vi "Tosca-Init AI Processing.vi"(0 "Queue data":T2) -> (4 "state":T1)   [LabVIEW 2020]
uses:
  Typedefs/Tosca-AI Control Queue Data.ctl
  Typedefs/Tosca-AI.ctl
  Typedefs/Tosca-AI Plot State.ctl
  epl-vi-lib/Connection VIs/Type Defs/CM-IO Type.ctl
  Sub VIs/Tosca-Globals.vi
  epl-vi-lib/Utility VIs/Array Manipulation VIs/Sort and Index (string).vi
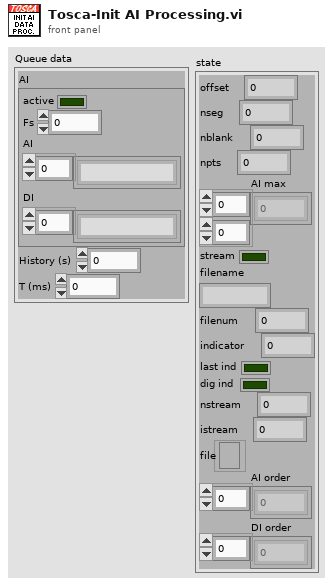
[diagram p1: front panel]
types:
  T1 = typedef "Tosca-AI Plot State.ctl" = cluster{"offset":i32, "nseg":i32, "nblank":i32, "npts":i32, "AI max":dbl[][], "stream":bool, "filename":string, "filenum":i32, "indicator":i32, "last ind":bool, "dig ind":bool, "nstream":i32, "istream":i32, "file":refnum<file>, "AI order":i32[], "DI order":i32[]}
  T2 = typedef "Tosca-AI Control Queue Data.ctl" = cluster{"AI":T3, "History (s)":dbl, "T (ms)":dbl}
  T3 = typedef "Tosca-AI.ctl" = cluster{"active":bool, "Fs":dbl, "AI":string[], "DI":string[]}
  T4 = typedef "CM-IO Type.ctl" = enum16{"Analog Outputs", "Analog Inputs", "Digital Outputs", "Digital Inputs"}
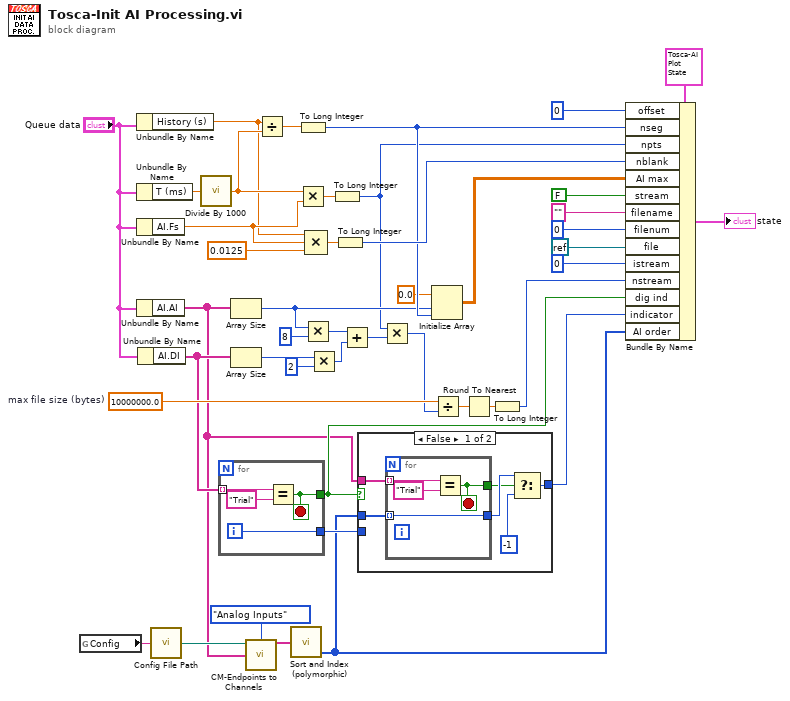
[diagram p0: block diagram]
diagram:
  w15 = 10000000.0  # max file size (bytes)
  n1 = global read "Tosca-Globals.vi" "Config"() -> (w1:string)
  n2 = Unbundle By Name("Queue data") -> ("History (s)"=w31:dbl)
  n3 = Unbundle By Name("Queue data") -> ("T (ms)"=w30:dbl)
  n4 = Unbundle By Name("Queue data") -> ("AI.Fs"=w39:dbl)
  n5 = Unbundle By Name("Queue data") -> ("AI.AI"=w3:string[])
  n6 = Unbundle By Name("Queue data") -> ("AI.DI"=w10:string[])
  n7 = call "Config File Path.vi"("AppName"=w1) -> ("Default config file name"=w6:path)
  n8 = call "Divide By 1000.vi"("X"=w30) -> ("X/1000"=w35:dbl)
  n9 = for {
    tunnel: w10 -> [w48] mode=indexing
    tunnel: [w46] -> w9
    tunnel: [w45] -> w7
    i -> [w46]
    stop <- w45 stop-if-true
    n10 = Equal?(x=w48, y="Trial") -> (x = y?=w45:bool)
  }
  n11 = Array Size(array=w3) -> (size(s)=w23:i32)
  n12 = Array Size(array=w10) -> (size(s)=w21:i32)
  n13 = call "CM-Endpoints to Channels.vi"("Path"=w6, "IO Type"=CM-IO_Type."Analog Inputs", "Requested Endpoints"=w3) -> ("IO Channels"=w4:string[])  [unwired: 11 in, 1 out]
  n14 = Divide(x=w31, y=w35) -> (x/y=w44:dbl)
  n15 = call-poly "Sort and Index (polymorphic).vi"("X"=w4) -> ("Index"=w2:i32[])  [unwired: 3 in, 1 out]
  n16 = To Long Integer(number=w44) -> (32bit integer=w34:i32)
  n17 = Multiply(x=w35, y=w39) -> (x*y=w41:dbl)
  n18 = Multiply(x=w23, y=8) -> (x*y=w19:i32)
  n19 = Compound Arithmetic op=MULTIPLY(w31, w39, 0.0125 ("y")) -> (w40:dbl)
  n20 = Multiply(x=w21, y=2) -> (x*y=w18:i32)
  n21 = To Long Integer(number=w41) -> (32bit integer=w16:i32)
  n22 = To Long Integer(number=w40) -> (32bit integer=w37:i32)
  n23 = Add(x=w19, y=w18) -> (x+y=w17:i32)
  n24 = case shown="False" w7 {
    tunnel: w9 -> [_ w59]
    tunnel: w3 -> [w54 _]
    tunnel: [w53 w59] -> w8
    tunnel: w2 -> [w49 _]
    frame False {
      n25 = for {
        tunnel: w54 -> [w58] mode=indexing
        tunnel: [w55] -> w52
        tunnel: [w56] -> w50
        tunnel: w49 -> [w55] mode=indexing
        stop <- w56 stop-if-true
        n26 = Equal?(x=w58, y="Trial") -> (x = y?=w56:bool)
      }
      n27 = Select(t=w52, s=w50, f=-1) -> (s? t:f=w53:i32)
    }
    frame True {
    }
  }
  n28 = Multiply(x=w16, y=w17) -> (x*y=w14:i32)
  n29 = Initialize Array(0.0 ("element"), w23, w34) -> (w32:dbl[][])
  n30 = Divide(x=w15, y=w14) -> (x/y=w13:dbl)
  n31 = Round To Nearest(number=w13) -> (nearest integer value=w12:dbl)
  n32 = To Long Integer(number=w12) -> (32bit integer=w11:i32)
  n33 = Bundle By Name(cluster=T1 {"offset"=0, "nseg"=0, "nblank"=0, "npts"=0, "AI max"=[], "stream"=FALSE, "filename"="", "filenum"=0, "indicator"=0, "last ind"=FALSE, "dig ind"=FALSE, "nstream"=0, "istream"=0, "file"=refnum, "AI order"=[], "DI order"=[]} ("state"), "offset"=0, "nseg"=w34, "npts"=w16, "nblank"=w37, "AI max"=w32, "stream"=FALSE, "filename"="" ("filestem"), "filenum"=0, "file"=refnum<k0> refnum, "istream"=0 ("nstream"), "nstream"=w11, "dig ind"=w7, "indicator"=w8, "AI order"=w2) -> (→"state":T1)
